vi "Event Loop.vi"(8 "Error Q":refnum<queue>, 9 "Helper Loop Q":refnum<queue>, 10 "Actor":refnum<class "Actor.lvclass">, 11 "Dev Actor Panel":refnum<class "Dev Panel.lvclass">) -> ()   [LabVIEW 2021, in "Dev Panel.lvclass"]
uses:
  Dev Panel.lvclass
  C:/git/jettl/src/temp/Helper Loop/Helper Loop.lvclass
  Actor/Actor/Actor.lvclass
  Helper Loop/Helper Loop.lvclass
  Dev Panel.lvclass/Dev Panel.ctl
  Actor/Msgs/Teardown/Teardown Msg/Teardown Msg.lvclass
  C:/git/jettl/src/Actor/Msg/Msg.lvclass
  Msgs/Pop Up/Pop Up Msg/Pop Up Msg.lvclass
  Actor/Msgs/Merge Error/Merge Error Msg/Merge Error Msg.lvclass
panel:
  in  "Button":bool
  out "String Indicator":string
  in  "Pop Up":bool
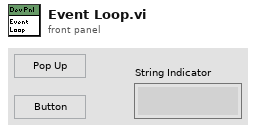
[diagram p1: front panel]
types:
  T1 = cluster{"Teardown":refnum<user-event>, "Pop Up":refnum<user-event>, "String Indicator":refnum<user-event>, "Button":refnum<user-event>}
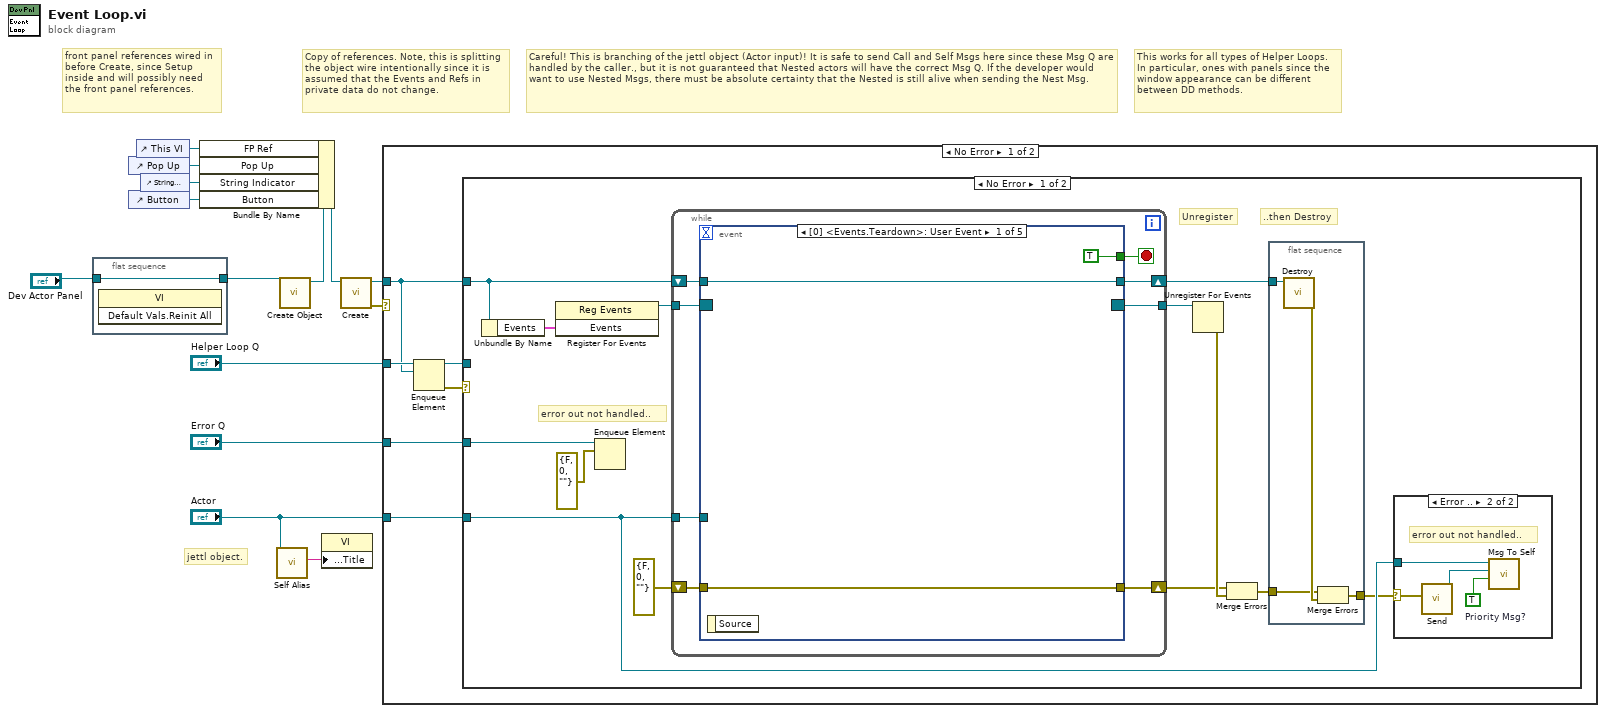
[diagram p0: block diagram]
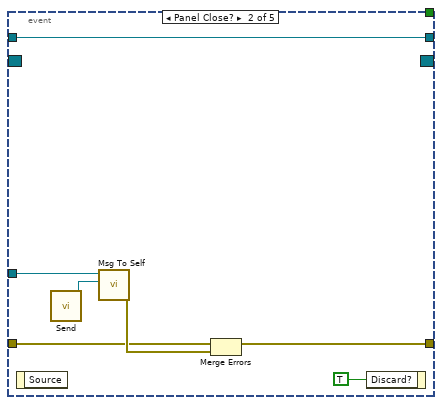
[diagram p3: hidden frame]
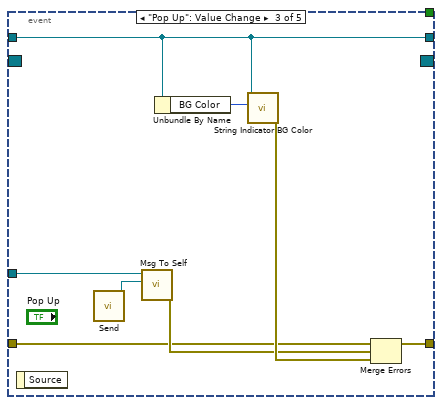
[diagram p4: hidden frame]
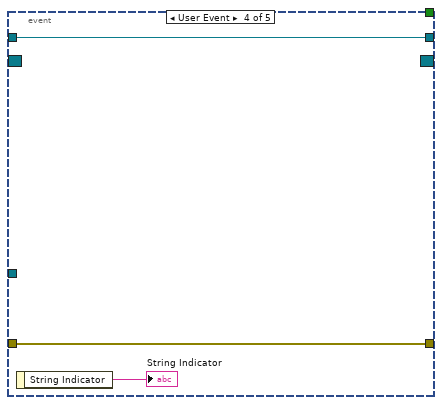
[diagram p5: hidden frame]
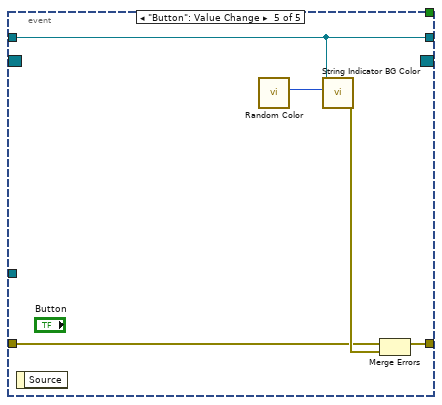
[diagram p6: hidden frame]
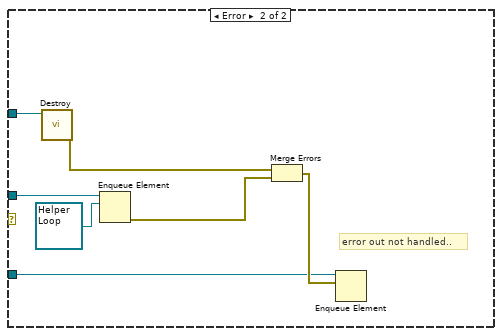
[diagram p7: hidden frame]
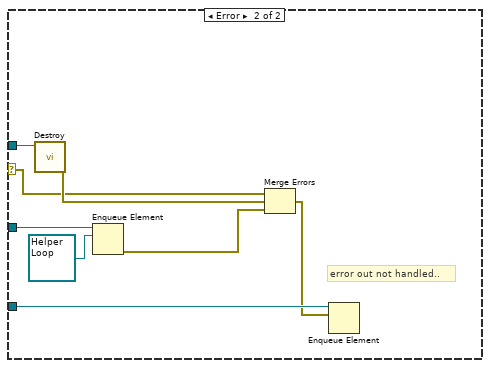
[diagram p8: hidden frame]
diagram:
  # "Copy of references. Note, this is splitting the object wire intentionally since it is assumed that the Events and Refs in private data do not change."
  # "front panel references wired in before Create, since Setup inside and will possibly need the front panel references."
  # "This works for all types of Helper Loops. In particular, ones with panels since the window appearance can be different between DD methods."
  # "jettl object."
  # "Careful! This is branching of the jettl object (Actor input)! It is safe to send Call and Self Msgs here since these Msg Q are handled by the caller., but it is not guaranteed that Nested actors will have the correct Msg Q. If the developer would want to use Nested Msgs, there must be absolute certainty that the Nested is still alive when sending the Nest Msg."
  n1 = flat-sequence {
    tunnel: [w15] -> w2
    tunnel: "Dev Actor Panel" -> [w15]
    frame #0 {
      n2 = invoke class="VI" method="Default Vals.Reinit All"() -> ()  [unwired: 3 in, 3 out]
    }
  }
  n3 = control-ref of="Pop Up"() -> (w12:refnum<vi>)
  n4 = control-ref of="Button"() -> (w11:refnum<vi>)
  n5 = control-ref of="This VI"() -> (w5:refnum<vi>)
  n6 = control-ref of="String Indicator"() -> (w13:refnum<vi>)
  n7 = call-dynamic "Self Alias.vi"("Actor in"="Actor") -> ("Alias"=w3:string)  [unwired: 9 in, 1 out]
  n8 = call "Create Object.vi"("Dev Panel in"=w2) -> ("Dev Panel out"=w6:refnum<class "Dev Panel.lvclass">)  [unwired: 10 in]
  n9 = Bundle By Name(cluster=w6, "FP Ref"=w5, "Pop Up"=w12, "String Indicator"=w13, "Button"=w11) -> (w7:refnum<class "Dev Panel.lvclass">)
  n10 = property class="VI"("Front Panel.Title"=w3) -> ()  [unwired: 2 in, 2 out]
  n11 = call "Create.vi"("Dev Actor Panel in"=w7) -> ("error out"=w14:errorcluster, "Dev Actor Panel out"=w8:refnum<class "Dev Panel.lvclass">)  [unwired: 9 in]
  n12 = case shown="No Error" w14 {
    selector: w14 -> [_ w89]
    tunnel: "Actor" -> [w21 _]
    tunnel: w8 -> [w18 w91]
    tunnel: "Error Q" -> [w20 w88]
    tunnel: "Helper Loop Q" -> [w19 w86]
    frame No Error {
      n13 = Enqueue Element(queue=w19, element=w18) -> (queue out=w16:refnum<queue>, error out=w17:errorcluster)  [unwired: 2 in, 1 out]
      n14 = case shown="No Error" w17 {
        tunnel: w21 -> [w34 _]
        tunnel: w20 -> [w24 w79]
        tunnel: w18 -> [w22 w77]
        tunnel: w16 -> [_ w78]
        frame No Error {
          # "error out not handled.."
          # "..then Destroy"
          # "Unregister"
          n15 = Unbundle By Name(w22) -> ("Events"=w31:T1)
          n16 = register-events ("Main Register for Events")(w31) -> (reference out=w32:refnum<event-registration>)  [unwired: 2 in, 1 out]
          n17 = Enqueue Element(queue=w24, element=errorcluster {"status"=FALSE, "code"=0, "source"=""}) -> ()  [unwired: 2 in, 3 out]
          n18 = while {
            tunnel: w34 -> [w47]
            shift-right: [w46] -> w27
            shift-left: w22 -> [w45]
            tunnel: w32 -> [w50]
            tunnel: [w48] -> w33
            shift-right: [w44] -> w28
            shift-left: errorcluster {"status"=FALSE, "code"=0, "source"=""} ("error out") -> [w43]
            stop <- w49 stop-if-true
            n19 = event "UI Events" shown="[0] <Events.Teardown>: User Event" {
              selector: w50 -> [_ _ _ _ _]
              dyn-events: [_ _ _ _ _] -> w48
              timeout: _ -> [_ _ _ _ _]
              tunnel: [TRUE _ _ _ _] -> w49
              tunnel: w47 -> [_ w59 w67 _ _]
              tunnel: [w52 w54 w62 w71 w76] -> w46
              tunnel: w45 -> [w52 w54 w62 w71 w76]
              tunnel: [w51 w56 w66 w70 w75] -> w44
              tunnel: w43 -> [w51 w57 w63 w70 w73]
              event User Event {
                n20 = event-data() -> ()  [unwired: 1 in, 1 out]
              }
              event Panel Close? {
                n21 = event-data() -> ()  [unwired: 1 in, 1 out]
                n22 = call "Send.vi"() -> ("Teardown Msg out"=w55:refnum<class "Teardown Msg.lvclass">)  [unwired: 11 in]
                n23 = call-dynamic "Msg To Self.vi"("Msg"=w55, "Actor in"=w59) -> ("error out"=w58:errorcluster)  [unwired: 9 in]
                n24 = Merge Errors(w57, w58) -> (w56:errorcluster)
                n25 = event-data("Discard?"=TRUE) -> ()  [unwired: 1 in, 1 out]
              }
              event "Pop Up": Value Change {
                n26 = event-data() -> ()  [unwired: 1 in, 1 out]
                n27 = call "Send.vi"() -> ("Pop Up Msg out"=w68:refnum<class "Pop Up Msg.lvclass">)  [unwired: 11 in]
                n28 = call-dynamic "Msg To Self.vi"("Msg"=w68, "Actor in"=w67) -> ("error out"=w64:errorcluster)  [unwired: 9 in]
                n29 = Unbundle By Name(w62) -> ("BG Color"=w61:u32)
                n30 = call "String Indicator BG Color.vi"("BG Color"=w61, "Dev Panel in"=w62) -> ("error out"=w65:errorcluster)  [unwired: 9 in]
                n31 = Merge Errors(w63, w64, w65) -> (w66:errorcluster)
              }
              event User Event {
                n32 = event-data() -> ("String Indicator"=→"String Indicator":string)  [unwired: 1 in]
              }
              event "Button": Value Change {
                n33 = event-data() -> ()  [unwired: 1 in, 1 out]
                n34 = call "Random Color.vi"() -> ("Color"=w72:u32)  [unwired: 11 in]
                n35 = call "String Indicator BG Color.vi"("BG Color"=w72, "Dev Panel in"=w76) -> ("error out"=w74:errorcluster)  [unwired: 9 in]
                n36 = Merge Errors(w73, w74) -> (w75:errorcluster)
              }
            }
          }
          n37 = Unregister For Events(event registration refnum=w33) -> (error out=w29:errorcluster)  [unwired: 1 in]
          n38 = Merge Errors(w28, w29) -> (w26:errorcluster)
          n39 = flat-sequence {
            tunnel: w27 -> [w42]
            tunnel: [w41] -> w25
            tunnel: w26 -> [w39]
            frame #0 {
              n40 = call "Destroy.vi"("Dev Actor Panel in"=w42) -> ("error out"=w40:errorcluster)  [unwired: 10 in]
              n41 = Merge Errors(w39, w40) -> (w41:errorcluster)
            }
          }
          n42 = case shown="Error .." w25 {
            selector: w25 -> [_ w36]
            tunnel: w34 -> [_ w38]
            frame No Error {
            }
            frame Error {
              w37 = TRUE  # Priority Msg?
              # "error out not handled.."
              n43 = call "Send.vi"("Error"=w36) -> ("Merge Error Msg out"=w35:refnum<class "Merge Error Msg.lvclass">)  [unwired: 10 in]
              n44 = call-dynamic "Msg To Self.vi"("Priority Msg?"=w37, "Msg"=w35, "Actor in"=w38) -> ()  [unwired: 8 in, 1 out]
            }
          }
        }
        frame Error {
          # "error out not handled.."
          n45 = call "Destroy.vi"("Dev Actor Panel in"=w77) -> ("error out"=w83:errorcluster)  [unwired: 10 in]
          n46 = Enqueue Element(queue=w78, element=refnum<class "Helper Loop.lvclass"> refnum) -> (error out=w80:errorcluster)  [unwired: 2 in, 2 out]
          n47 = Merge Errors(w83, w80) -> (w82:errorcluster)
          n48 = Enqueue Element(queue=w79, element=w82) -> ()  [unwired: 2 in, 3 out]
        }
      }
    }
    frame Error {
      # "error out not handled.."
      n49 = call "Destroy.vi"("Dev Actor Panel in"=w91) -> ("error out"=w90:errorcluster)  [unwired: 10 in]
      n50 = Enqueue Element(queue=w86, element=refnum<class "Helper Loop.lvclass"> refnum) -> (error out=w84:errorcluster)  [unwired: 2 in, 2 out]
      n51 = Merge Errors(w89, w90, w84) -> (w87:errorcluster)
      n52 = Enqueue Element(queue=w88, element=w87) -> ()  [unwired: 2 in, 3 out]
    }
  }
